vi "Thermistor Read.vi"(0 "Arduino Resource":T1={"VISA resource"="COM11", "Board Type"=enum."Uno", "Connection Type"=enum."USB / Serial", "Bytes Per Packet (15)"=15}, 1 "Units (C)":enum16{"Celsius", "Fahrenheit", "Kelvin"}(ring), 5 "Thermistor AI Pin (0)":u8, 7 "Paired Resistance (10K Ohms)":dbl=10000.0, 9 "Vcc (5 v)":dbl=5.0, 11 "error in":errorcluster) -> (4 "Arduino Resource":T1={"VISA resource"="COM11", "Board Type"=enum."Uno", "Connection Type"=enum."USB / Serial", "Bytes Per Packet (15)"=15}, 8 "Temperature":dbl, 15 "error out":errorcluster)   [LabVIEW 2015, in "LabVIEW Interface for Arduino.lvlib"]
doc: "Read the temperature from a thermistor. Thermistor must be used in a voltage divider with a paired resistance. The paired resistance is user selectable however a value of 10K Ohms is recommended."
uses:
  <vilib>/LabVIEW Interface for Arduino/LabVIEW Interface for Arduino.lvlib
  <vilib>/LabVIEW Interface for Arduino/Type Defs/Arduino Resource.ctl
  <vilib>/LabVIEW Interface for Arduino/Type Defs/Board Type.ctl
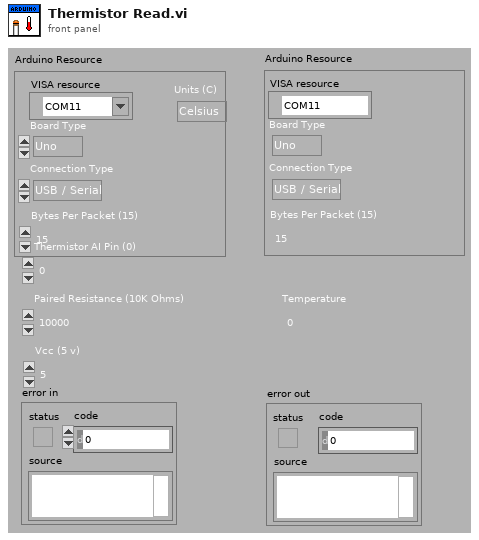
[diagram p1: front panel]
types:
  T1 = typedef "LabVIEW Interface for Arduino.lvlib/Arduino Resource.ctl" = cluster{"VISA resource":refnum<visa-resource-name>, "Board Type":T2, "Connection Type":enum8{"USB / Serial"}, "Bytes Per Packet (15)":u8}
  T2 = typedef "LabVIEW Interface for Arduino.lvlib/Board Type.ctl" = enum16{"Uno", "Dimuelanove w/Atmega 328", "Mega 2560"}
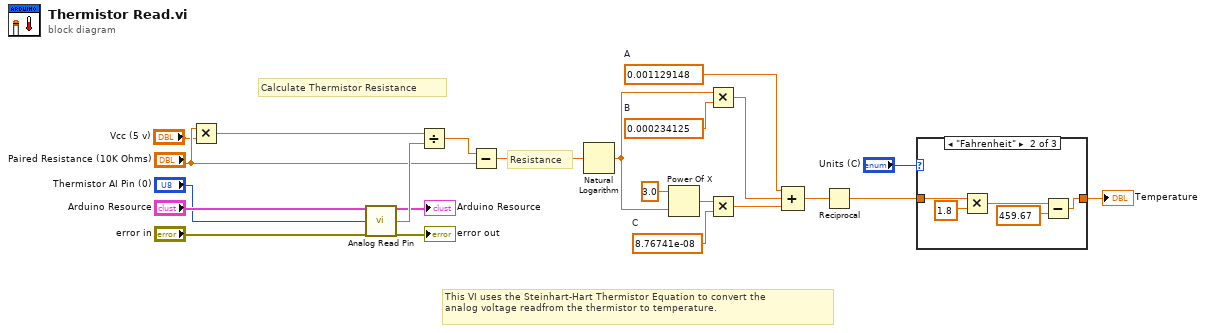
[diagram p0: block diagram]
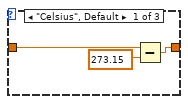
[diagram p2: hidden frame]
diagram:
  w17 = 8.76741e-08  # C
  w14 = 0.001129148  # A
  w19 = 0.000234125  # B
  # "Resistance"
  # "This VI uses the Steinhart-Hart Thermistor Equation to convert the \nanalog voltage readfrom the thermistor to temperature."
  # "Calculate Thermistor Resistance"
  n1 = Multiply(x="Paired Resistance (10K Ohms)", y="Vcc (5 v)") -> (x*y=w23:dbl)
  n2 = call <vilib>:"Analog Read Pin.vi"("Arduino Resource"="Arduino Resource", "Analog Input Pin (0)"="Thermistor AI Pin (0)", "error in"="error in") -> ("Arduino Resource"=→"Arduino Resource":T1, "Voltage"=w22:dbl, "error out"=→"error out":errorcluster)  [unwired: 10 in]
  n3 = Divide(x=w23, y=w22) -> (x/y=w21:dbl)
  n4 = Subtract(x=w21, y="Paired Resistance (10K Ohms)") -> (x-y=w20:dbl)
  n5 = Natural Logarithm(1:w20) -> (0:w5:dbl)
  n6 = Power Of X(1:w5, 2:3.0 ("x")) -> (0:w18:dbl)
  n7 = Multiply(x=w5, y=w19) -> (x*y=w15:dbl)
  n8 = Multiply(x=w18, y=w17) -> (x*y=w16:dbl)
  n9 = Compound Arithmetic op=ADD(w14, w15, w16) -> (w13:dbl)
  n10 = Reciprocal(x=w13) -> (1/x=w12:dbl)
  n11 = case shown="\"Fahrenheit\"" "Units (C)" {
    tunnel: w12 -> [w26 w31 w32]
    tunnel: [w24 w27 w32] -> w4
    frame "Celsius", Default {
      n12 = Subtract(x=w26, y=273.15) -> (x-y=w24:dbl)
    }
    frame "Fahrenheit" {
      n13 = Multiply(x=w31, y=1.8) -> (x*y=w29:dbl)
      n14 = Subtract(x=w29, y=459.67) -> (x-y=w27:dbl)
    }
    frame "Kelvin" {
    }
  }
  "Temperature" <- w4
